vi "Get Relation Definition.vi"(11 "Relation in":refnum<class "Relation.lvclass">) -> (2 "Relation":T1)   [LabVIEW 2020, in "Conditum.lvlib" / "Columns.lvlib" / "Relation.lvclass"]
uses:
  Relation.lvclass
  Relation Info.ctl
  Relation Mapping.ctl
  Relation.lvclass/Relation.ctl
  Conditum.lvlib
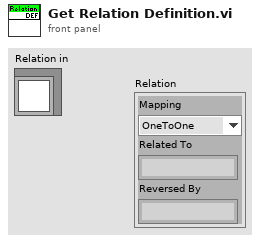
[diagram p1: front panel]
types:
  T1 = typedef "Conditum.lvlib/Relation Info.ctl" = cluster{"Mapping":T2, "Related To":string, "Reversed By":string}
  T2 = typedef "Conditum.lvlib/Relation Mapping.ctl" = enum16{"OneToOne", "OneToMany", "ManyToOne", "ManyToMany"}
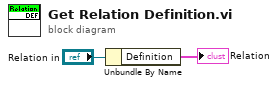
[diagram p0: block diagram]
diagram:
  n1 = Unbundle By Name("Relation in") -> ("Definition"=→"Relation":T1)
